vi "real time object tracker v1.1 EJA 09 14 2016.vi"() -> ()   [LabVIEW 2015]
doc: "The Low-Level Grab VI acquires images continuously and displays the images in an image control using low-level acquisition VIs. A grab is appropriate for high-speed applications in which you need to process only one image at a time."
uses:
  <vilib>/userdefined/High Color/IMAQdx.ctl
  <vilib>/vision/driver/IMAQdx.llb/IMAQdx Buffer Number Mode.ctl
  <vilib>/vision/driver/NI_Vision_Acquisition_Software.lvlib
  <resource>/objmgr/imaqdx.rc
panel:
  out "time vs iteration":cluster{dbl[], i32[]}(graph)
  out "FPS":i32=42
  out "time (s)":dbl[](array[numeric]) format="%.3f"
  in  "Origin":cluster{"X":i32, "Y":i32}
  out "Y position vs time":cluster{dbl[], i32[]}(graph)
  out "X position vs time":cluster{dbl[], i32[]}(graph)
  in  "threshhold":i32=221
  out "found\nedge\nin ROI":bool[](array[boolean])
  in  "image row min":i32=50
  in  "image row max":i32=1150
  in  "image col min":i32=50
  in  "image col max":i32=1900
  out "X positions\n(image \ncoordinates)":i32[](array[numeric])
  out "Y positions \n(image \ncoordinates)":i32[](array[numeric])
  out "LIVE":bool
  in  "stop":bool
  out "Backlog":i32(slide)=-1 scale=0.0..50.0
  in  "IMAQdx Device":T1="cam0"
  in  "Buffers":u32=50
  out "Image":T2(plugin-control)
  # "INSTRUCTIONS\n\nThis program finds the \ndarkest searching from\nright to left in an image.\nUsed to find trailing\nedge position of a\nswimming fish. Dark fish\non a light background.\n\nCan also be modified to \nfind lightest."
  # "issues\n\nHow do we know if frames \nare dropped?\n\nProbably will need to save data\nin sections to an open file\n\nCould have a sliding ROI based\non previous trailing edge position\n\nCould process each data chunk\nseparately to avoid frame dropping\nissues.  I.e. if you write every 1000\npoints, then in post processing only\nprocess 1000 at a time."
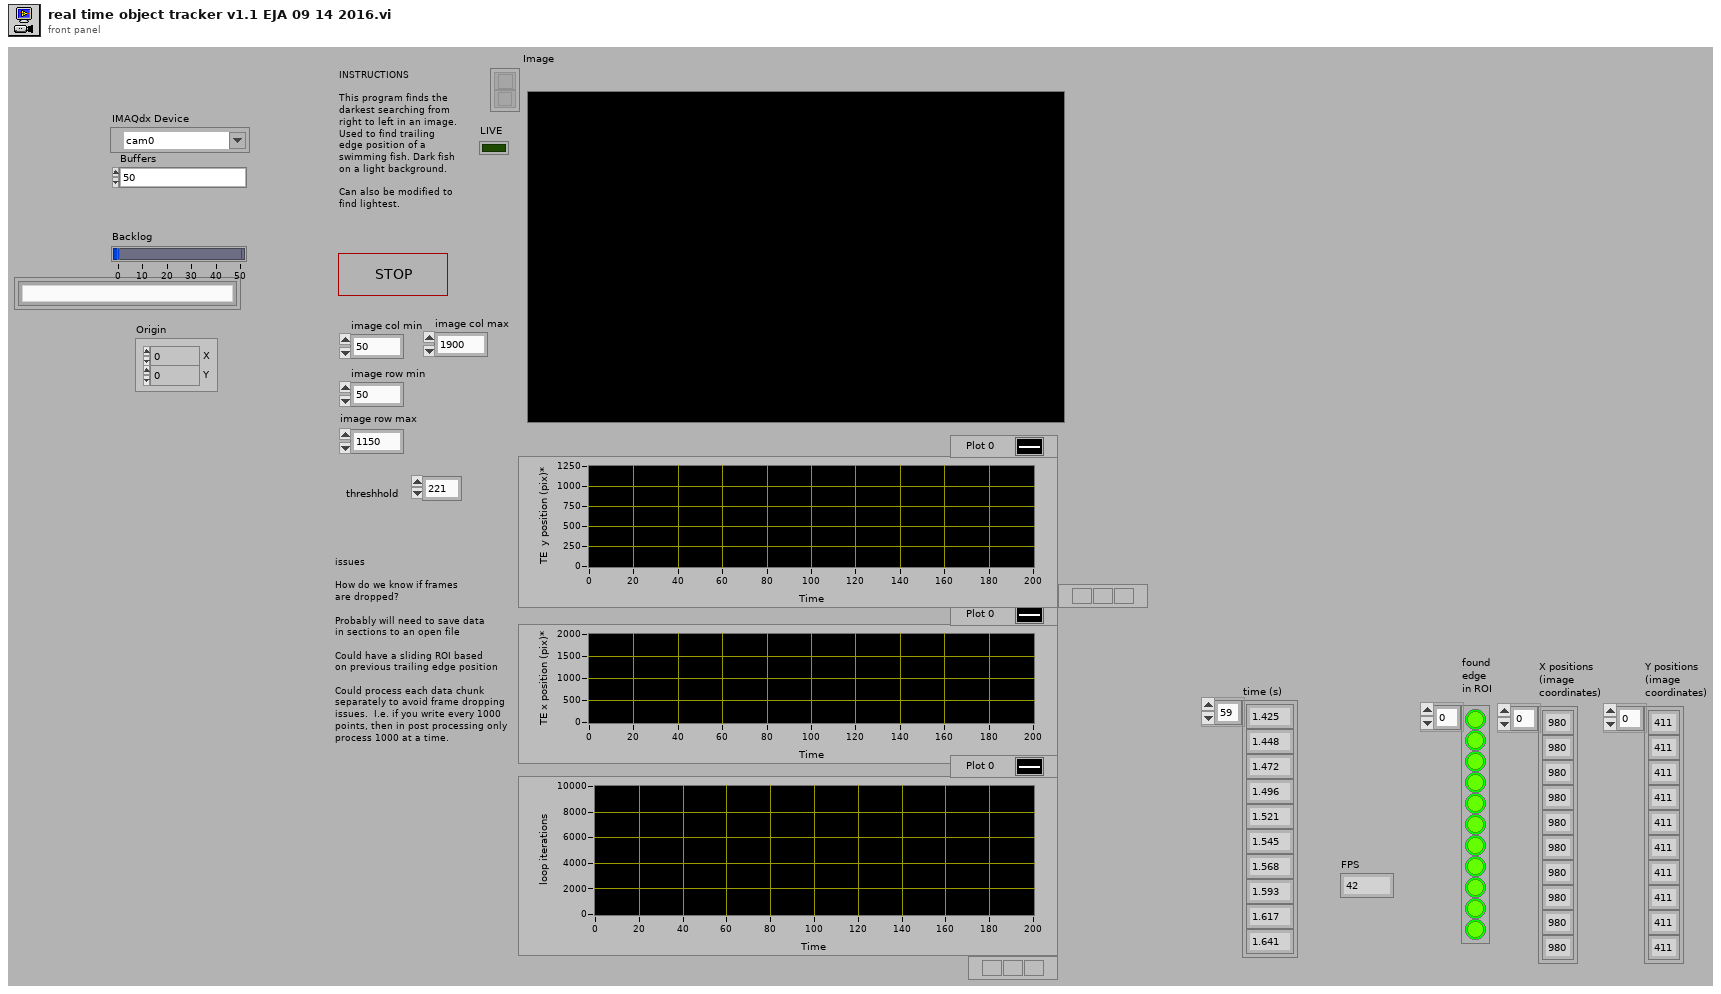
[diagram p1: front panel]
types:
  T1 = typedef "IMAQdx.ctl" = refnum<k21>
  T2 = typedef "IMAQ Image.ctl" = refnum<image>
  T3 = typedef "NI_Vision_Acquisition_Software.lvlib/IMAQdx Buffer Number Mode.ctl" = enum32{"Next", "Last", "Buffer Number", "Every", "Last New"}
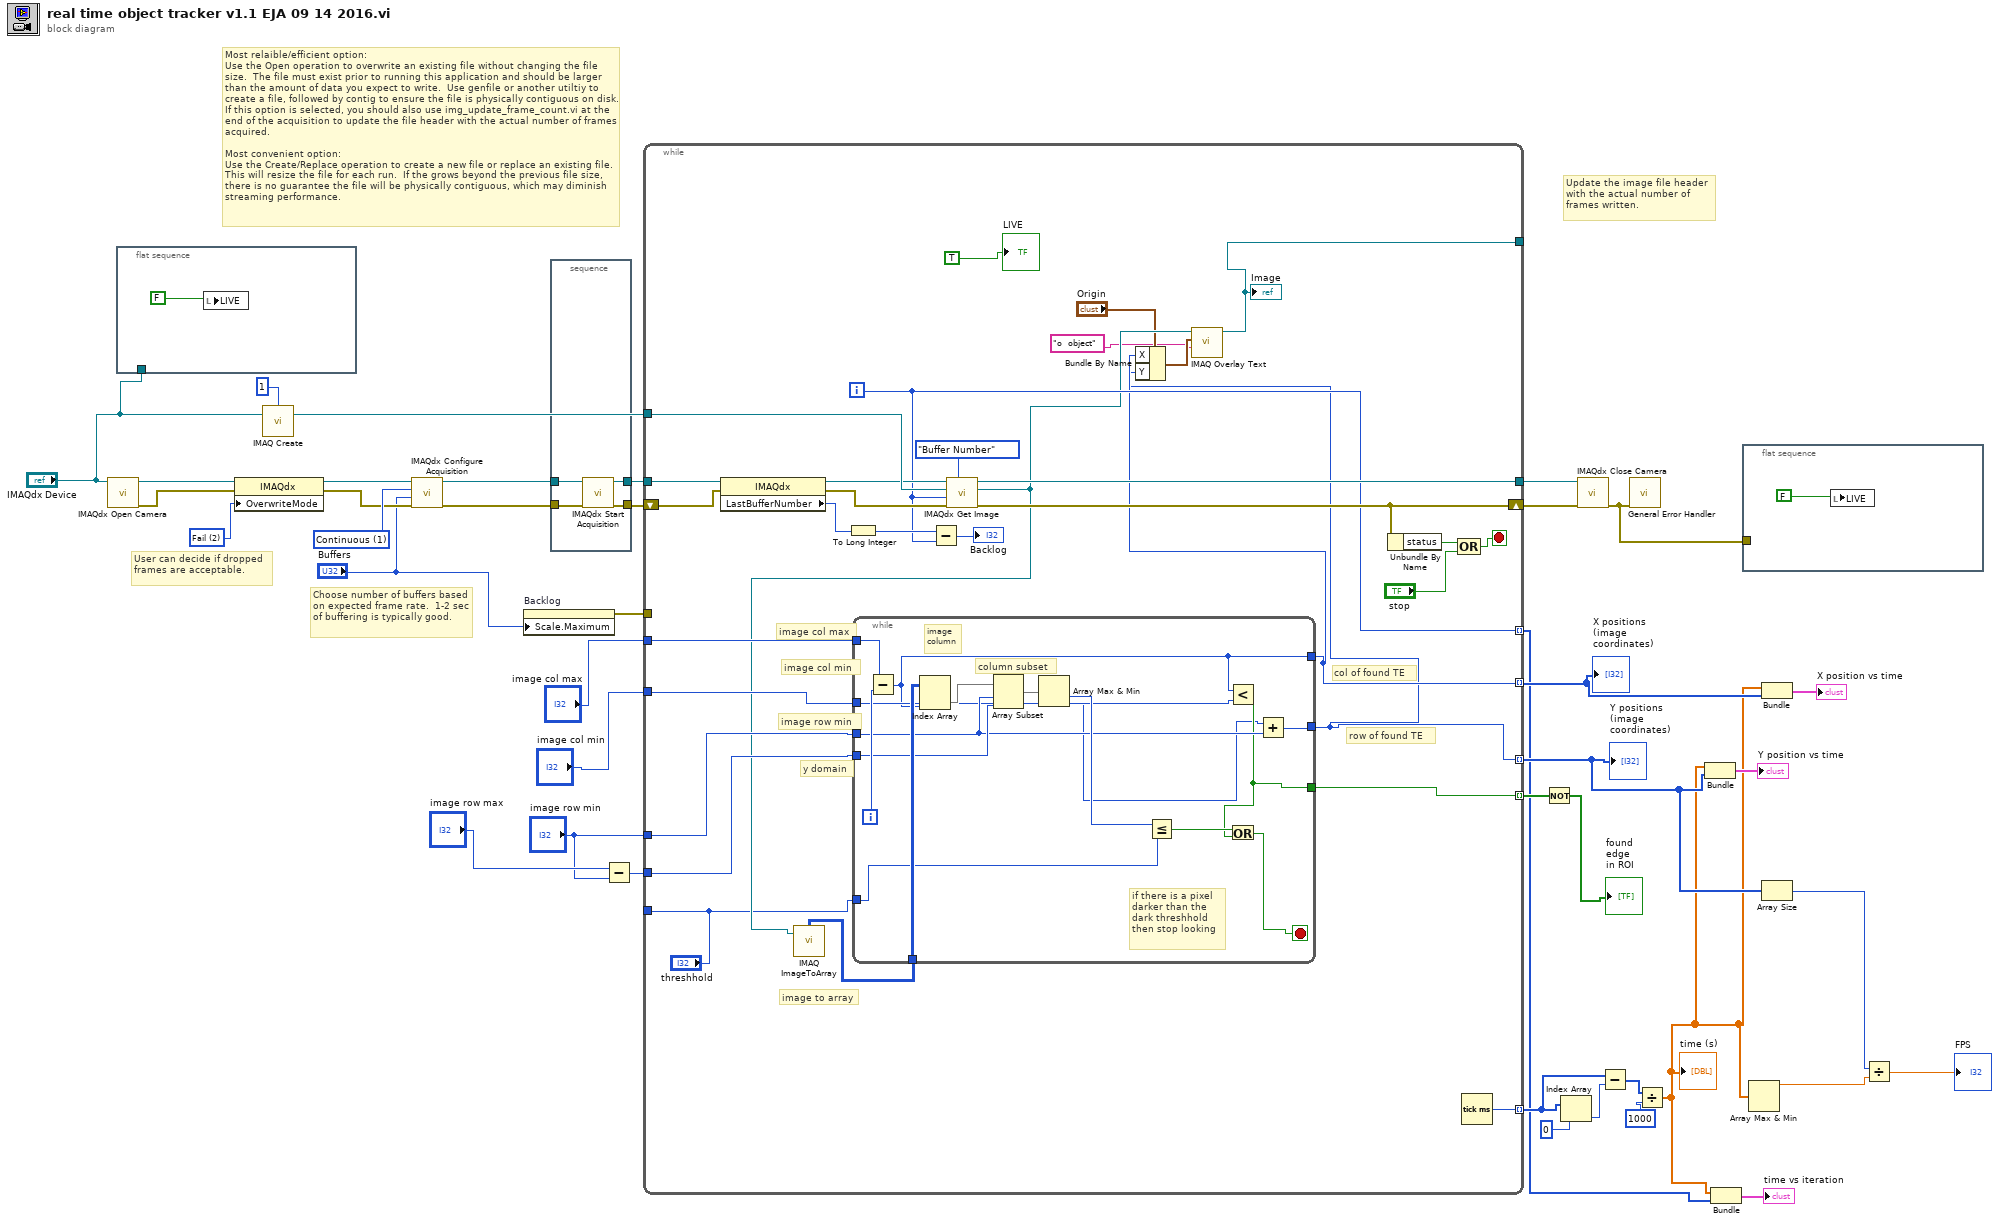
[diagram p0: block diagram]
diagram:
  w33 = u32 2 items=["Get Oldest"=0, "Fail"=2, "Get Newest"=3] ("OverwriteMode")
  w39 = u32 1 items=["One Shot", "Continuous"] ("Continuous ?")
  # "Update the image file header with the actual number of frames written."
  # "Choose number of buffers based on expected frame rate.  1-2 sec of buffering is typically good."
  # "User can decide if dropped frames are acceptable."
  # "Most relaible/efficient option:\nUse the Open operation to overwrite an existing file without changing the file size.  The file must exist prior to running this application and should be larger than the amount of data you expect to write.  Use genfile or another utiltiy to create a file, followed by contig to ensure the file is physically contiguous on disk.  If this option is selected, you should also use img_update_frame_count.vi at the end of the acquisition to update the file header with the actual number of frames acquired. \n\nMost convenient option:\nUse the Create/Replace operation to create a new file or replace an existing file. This will resize the file for each run.  If the grows beyond the previous file size, there is no guarantee the file will be physically contiguous, which may diminish streaming performance."
  n1 = call <vilib>:"IMAQdx Open Camera.vi"("Session In"="IMAQdx Device") -> ("error out"=w29:errorcluster, "Session Out"=w28:T1)  [unwired: 2 in, 7 out]
  n2 = flat-sequence {
    tunnel: "IMAQdx Device" -> [_]
    frame #0 {
      n3 = local write "LIVE"(FALSE) -> ()
    }
  }
  n4 = property class="IMAQdx"(reference=w28, error in=w29, "OverwriteMode"=w33) -> (reference out=w31:T1, error out=w30:errorcluster)
  n5 = call "IMAQ Create"("Border Size"=1, "Image Name"="IMAQdx Device") -> ("New Image"=w40:T2)  [unwired: 2 in, 2 out]
  n6 = call <vilib>:"IMAQdx Configure Acquisition.vi"("error in"=w30, "Number of Buffers"="Buffers", "Continuous?"=w39, "Session In"=w31) -> ("error out"=w25:errorcluster, "Session Out"=w32:T1)  [unwired: 6 out]
  n7 = property on="Backlog" class="Slide (strict)"("Scale.Maximum"="Buffers") -> (error out=w27:errorcluster)  [unwired: 2 in, 1 out]
  n8 = stacked-sequence {
    tunnel: [w45] -> w38
    tunnel: [w44] -> w37
    tunnel: w32 -> [w43]
    tunnel: w25 -> [w42]
    frame #0 {
      n9 = call <vilib>:"IMAQdx Start Acquisition.vi"("error in"=w42, "Session In"=w43) -> ("error out"=w45:errorcluster, "Session Out"=w44:T1)  [unwired: 8 out]
    }
  }
  n10 = Subtract(x="image row max", y="image row min") -> (x-y=w18:i32)
  n11 = while {
    tunnel: [w71] -> w35
    tunnel: w37 -> [w74]
    tunnel: w40 -> [w72]
    tunnel: [w53] -> _
    shift-right: [w70] -> w34
    shift-left: w38 -> [w73]
    tunnel: w27 -> [_]
    tunnel: "image col max" -> [w60]
    tunnel: "image col min" -> [w59]
    tunnel: "image row min" -> [w58]
    tunnel: w18 -> [w57]
    tunnel: ["threshhold"] -> _
    tunnel: [w51] -> w15 mode=indexing
    tunnel: [w50] -> w8 mode=indexing
    tunnel: [w56] -> w17 mode=indexing
    tunnel: [w55] -> w2 mode=indexing
    tunnel: [w47] -> w10 mode=indexing
    i -> [w55]
    stop <- w76 stop-if-true
    # "image col min"
    # "image col max"
    # "image row min"
    # "row of found TE"
    # "col of found TE"
    # "y domain"
    # "image to array"
    n12 = property class="IMAQdx"(reference=w74, error in=w73) -> (reference out=w67:T1, error out=w68:errorcluster, "LastBufferNumber"=w64:u32)
    n13 = To Long Integer(number=w64) -> (32bit integer=w63:i32)
    n14 = Subtract(x=w63, y=w55) -> (x-y=→"Backlog":i32)
    n15 = call <vilib>:"IMAQdx Get Image.vi"("Buffer Number Mode (Next)"=IMAQdx_Buffer_Number_Mode."Buffer Number", "error in"=w68, "Buffer Number In"=w55, "Image In"=w72, "Session In"=w67) -> ("error out"=w70:errorcluster, "Image Out"=w54:T2, "Session Out"=w71:T1)  [unwired: 1 in, 3 out]
    n16 = call "IMAQ ImageToArray"("Image"=w54) -> ("Image Pixels (U8)"=w61:u8[][])  [unwired: 2 in, 5 out]
    n17 = while {
      tunnel: w58 -> [w84]
      tunnel: [w82] -> w51
      tunnel: [w85] -> w50
      tunnel: w57 -> [w87]
      tunnel: w61 -> [w89]
      tunnel: w60 -> [w92]
      tunnel: w59 -> [w83]
      tunnel: [w79] -> w56
      tunnel: "threshhold" -> [w77]
      i -> [w91]
      stop <- w80 stop-if-true
      # "if there is a pixel\ndarker than the\ndark threshhold\nthen stop looking"
      # "column subset"
      # "image\ncolumn"
      n18 = Subtract(x=w92, y=w91) -> (x-y=w82:i32)
      n19 = Index Array(array=w89, index (col)=w82) -> (element=w88:u8[])  [unwired: 1 in]
      n20 = Array Subset(array=w88, index=w84, length=w87) -> (w86:u8[])
      n21 = Array Max & Min(array=w86) -> (min value=w90:u8, min index (indices)=w78:i32)  [unwired: 2 out]
      n22 = Less Or Equal?(x=w90, y=w77) -> (x <= y?=w81:bool)
      n23 = Less?(x=w82, y=w83) -> (x < y?=w79:bool)
      n24 = Or(x=w81, y=w79) -> (x .or. y?=w80:bool)
      n25 = Add(x=w78, y=w84) -> (x+y=w85:i32)
    }
    n26 = Bundle By Name(cluster="Origin", "X"=w51, "Y"=w50) -> (w49:cluster{"X":i32, "Y":i32})
    n27 = call "IMAQ Overlay Text"("String"="o  object", "Origin"=w49, "Image"=w54) -> ("Image Out"=w53:T2)  [unwired: 5 in, 3 out]
    "Image" <- w53
    n28 = Unbundle By Name(w70) -> ("status"=w75:bool)
    n29 = Compound Arithmetic op=OR(w75, "stop") -> (w76:bool)
    n30 = Tick Count (ms)() -> (millisecond timer value=w47:u32)
    "LIVE" <- TRUE
  }
  "X positions\n(image \ncoordinates)" <- w15
  "Y positions \n(image \ncoordinates)" <- w8
  n31 = Not(x=w17) -> (.not. x?=→"found\nedge\nin ROI":bool[])
  n32 = Index Array(array=w10, index=0) -> (element=w11:u32)
  n33 = call <vilib>:"IMAQdx Close Camera.vi"("error in"=w34, "Session In"=w35) -> ("error out"=w24:errorcluster)  [unwired: 9 out]
  n34 = Subtract(x=w10, y=w11) -> (x-y=w3:u32[])
  n35 = call <vilib>:"General Error Handler.vi"("error in (no error)"=w24) -> ()  [unwired: 2 in, 13 out]
  n36 = Divide(x=w3, y=1000) -> (x/y=w1:dbl[])
  "time (s)" <- w1
  n37 = Bundle(w1, w8) -> (→"Y position vs time":cluster{dbl[], i32[]})  [unwired: 1 out]
  n38 = Bundle(w1, w2) -> (→"time vs iteration":cluster{dbl[], i32[]})  [unwired: 1 out]
  n39 = flat-sequence {
    tunnel: w24 -> [_]
    frame #0 {
      n40 = local write "LIVE"(FALSE) -> ()
    }
  }
  n41 = Array Max & Min(array=w1) -> (max value=w9:dbl)  [unwired: 3 out]
  n42 = Bundle(w1, w15) -> (→"X position vs time":cluster{dbl[], i32[]})  [unwired: 1 out]
  n43 = Array Size(array=w8) -> (size(s)=w7:i32)
  n44 = Divide(x=w7, y=w9) -> (x/y=→"FPS":dbl)
